vi "AWGN.vi"(10 "AWGN (dB)":dbl(slide)=0.6 caption="Standard deviation" scale=-20.0..30.0, 11 "Dynamic Data":dynamicdata(waveform)) -> (3 "DC with Gaussian Noise":dynamicdata(waveform))   [LabVIEW 2013]
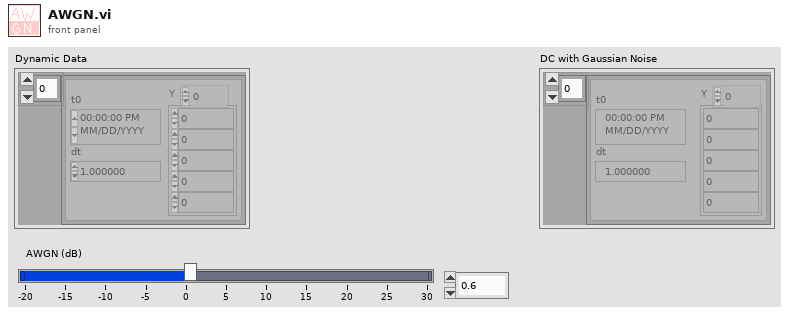
[diagram p1: front panel]
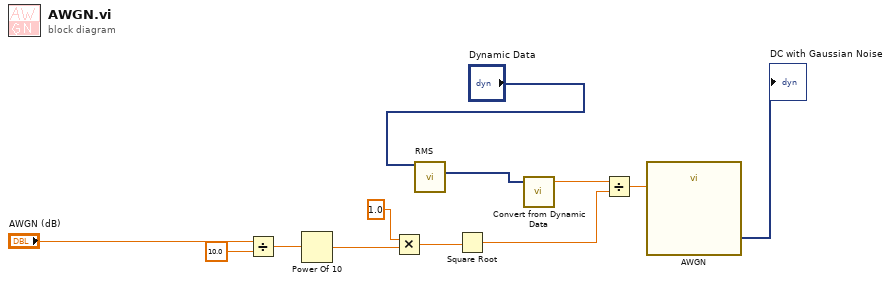
[diagram p0: block diagram]
diagram:
  n1 = Divide(x="AWGN (dB)", y=10.0) -> (x/y=w3:dbl)
  n2 = Power Of 10(x=w3) -> (10^x=w4:dbl)
  n3 = Multiply(x=1.0, y=w4) -> (x*y=w6:dbl)
  n4 = call "RMS"("Signals"="Dynamic Data") -> ("RMS"=w7:dynamicdata)  [unwired: 13 in, 1 out]
  n5 = Square Root(x=w6) -> (sqrt(x)=w9:dbl)
  n6 = call "Convert from Dynamic Data"("Dynamic Data Type"=w7) -> ("Scalar"=w8:dbl)  [unwired: 3 in]
  n7 = Divide(x=w8, y=w9) -> (x/y=w12:dbl)
  n8 = call "AWGN"("Standard deviation"=w12) -> ("DC with Gaussian Noise"=→"DC with Gaussian Noise":dynamicdata)  [unwired: 13 in, 1 out]
